vi "GEN_Initialize Path Constant.vi"(8 "error in":errorcluster, 11 "Path in":path) -> (0 "error out":errorcluster, 1 "File not exists?":bool caption="文件不存在", 2 "Path Constant":T1, 3 "Path dup":path)   [LabVIEW 2016]
uses:
  Sys Paths.ctl
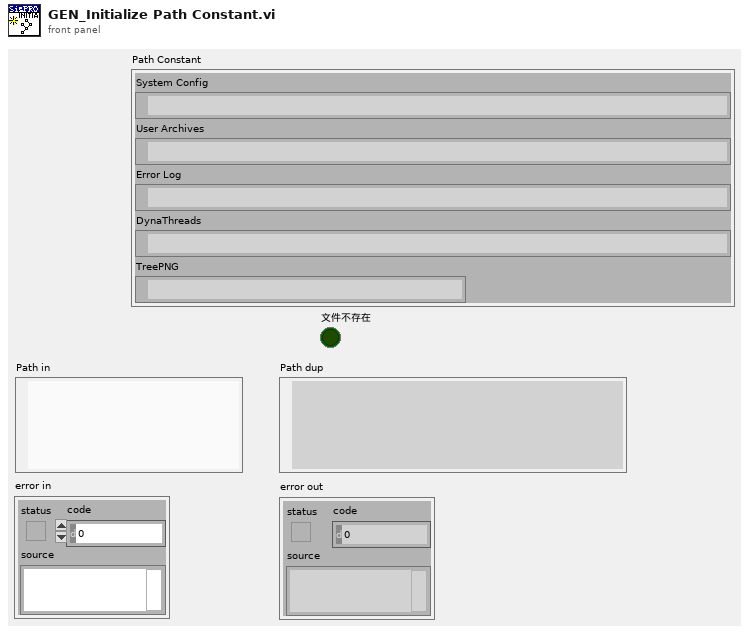
[diagram p1: front panel]
types:
  T1 = typedef "Sys Paths.ctl" = cluster{"System Config":path, "User Archives":path, "Error Log":path, "DynaThreads":path, "TreePNG":path}
  T2 = enum32{"invalid app kind", "Development System", "Run Time System", "Student Edition", "Embedded LabVIEW", "Evaluation", "Custom"}
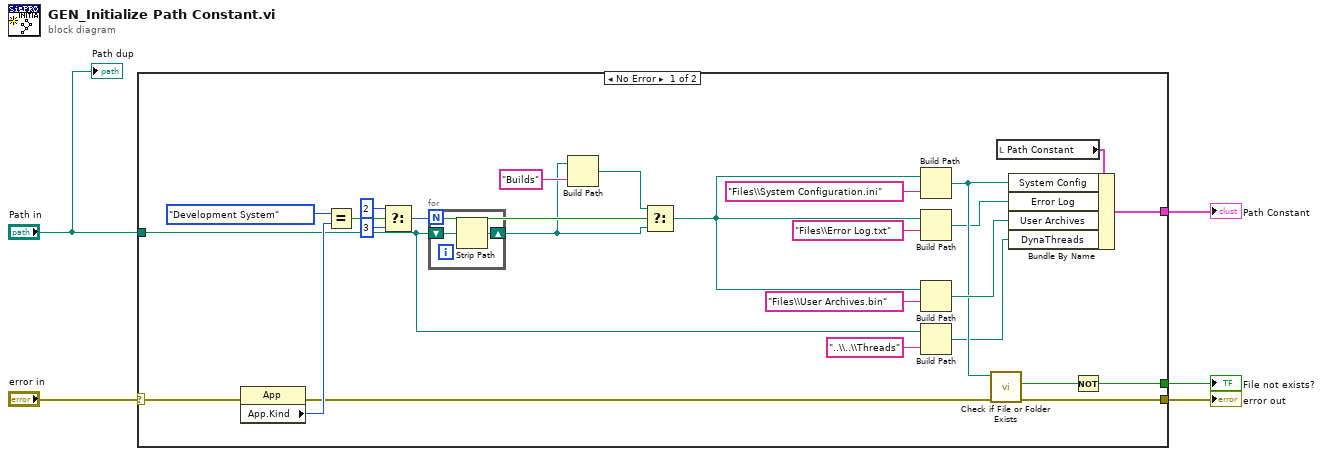
[diagram p0: block diagram]
diagram:
  n1 = case shown="No Error" "error in" {
    selector: "error in" -> [w24 w34]
    tunnel: "Path in" -> [w11 _]
    tunnel: [w25 _] -> w4
    tunnel: [w18 w34] -> w2
    tunnel: [w16 _] -> w1
    frame No Error {
      n2 = property class="App"(error in=w24) -> (error out=w19:errorcluster, "App.Kind"=w29:T2)  [unwired: 1 in, 1 out]
      n3 = Equal?(x=T2."Development System" ("y"), y=w29) -> (x = y?=w9:bool)
      n4 = Select(t=2 ("Times"), s=w9, f=3 ("Times")) -> (s? t:f=w14:i32)
      n5 = for {
        N: w14 -> [_]
        shift-right: [w32] -> w7
        shift-left: w11 -> [w33]
        n6 = Strip Path(path=w33) -> (stripped path=w32:path)  [unwired: 1 out]
      }
      n7 = Build Path(base path=w7, name or relative path="Builds") -> (appended path=w8:path)
      n8 = Select(t=w8, s=w9, f=w7) -> (s? t:f=w6:path)
      n9 = Build Path(base path=w6, name or relative path="Files\\System Configuration.ini") -> (appended path=w20:path)
      n10 = Build Path(base path=w6, name or relative path="Files\\Error Log.txt") -> (appended path=w13:path)
      n11 = Build Path(base path=w6, name or relative path="Files\\User Archives.bin") -> (appended path=w21:path)
      n12 = Build Path(base path=w11, name or relative path="..\\..\\Threads") -> (appended path=w12:path)
      n13 = call <vilib>:"Check if File or Folder Exists.vi"("error in (no error)"=w19, "path"=w20) -> ("error out"=w18:errorcluster, "file or folder exists?"=w17:bool)  [unwired: 7 in, 1 out]
      n14 = local read "Path Constant"() -> (w15:T1)
      n15 = Bundle By Name(cluster=w15, "System Config"=w20, "Error Log"=w13, "User Archives"=w21, "DynaThreads"=w12) -> (w25:T1)
      n16 = Not(x=w17) -> (.not. x?=w16:bool)
    }
    frame Error {
    }
  }
  "Path Constant" <- w4
  "error out" <- w2
  "File not exists?" <- w1
  "Path dup" <- "Path in"
